vi "day2-1.vi"() -> ()   [LabVIEW 2021]
uses:
  <vilib>/Utility/file.llb/Read Delimited Spreadsheet (string).vi
panel:
  in  "Example":string="A Y\nB X\nC Z"
  in  "Example":bool
  out "Answer":i64=10624
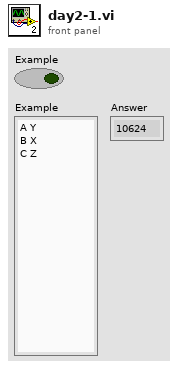
[diagram p1: front panel]
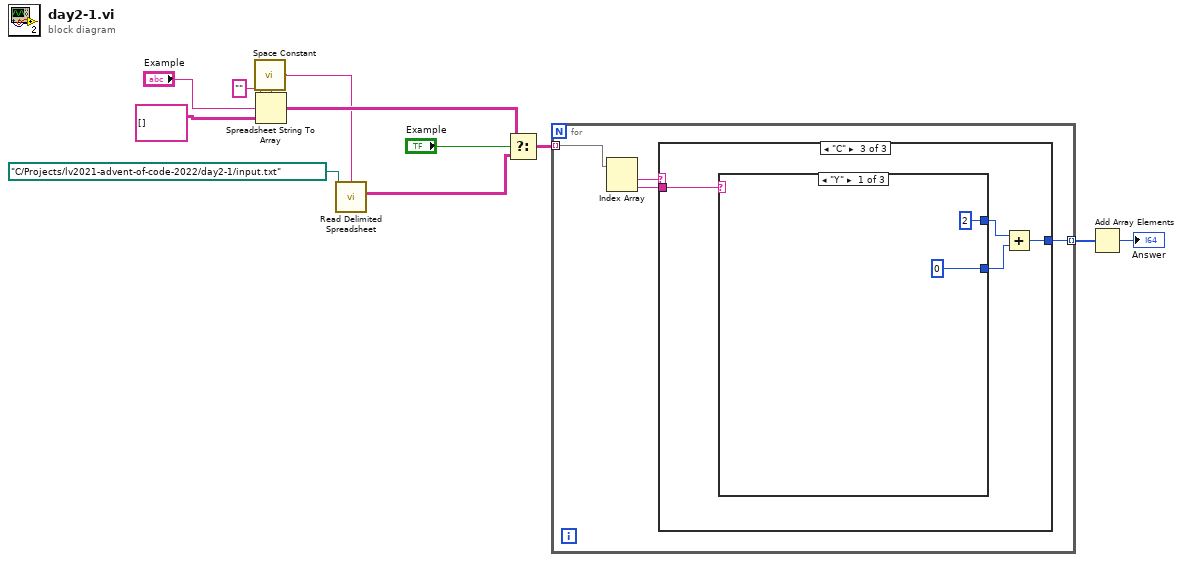
[diagram p0: block diagram]
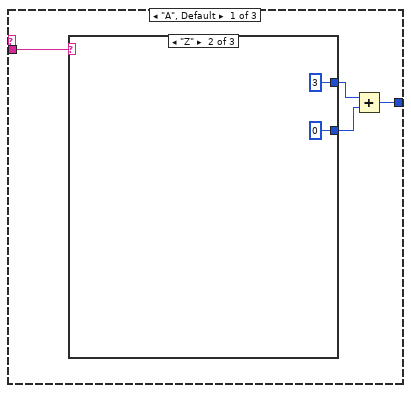
[diagram p2: hidden frame]
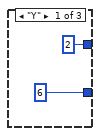
[diagram p3: hidden frame]
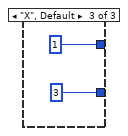
[diagram p4: hidden frame]
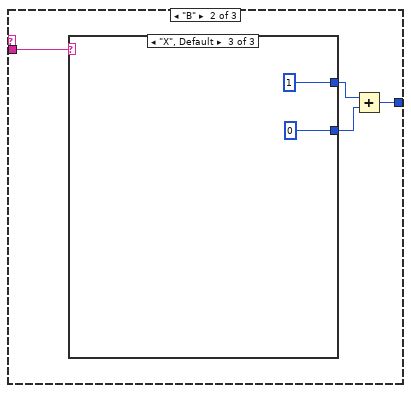
[diagram p5: hidden frame]
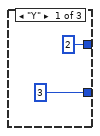
[diagram p6: hidden frame]
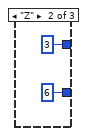
[diagram p7: hidden frame]
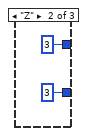
[diagram p8: hidden frame]
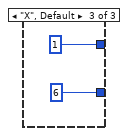
[diagram p9: hidden frame]
diagram:
  n1 = call <vilib>:"Space Constant.vi"() -> ("String"=w3:string)
  n2 = Spreadsheet String To Array(delimiter (Tab)=w3, format string="", spreadsheet string="Example", array type (2D Dbl)=string[][] [] ("t")) -> (array=w7:string[][])
  n3 = call-poly <vilib>:"Read Delimited Spreadsheet.vi"("file path (dialog if empty)"=path "C:/Projects/lv2021-advent-of-code-2022/day2-1/input.txt", "delimiter (\\t)"=w3) -> ("all rows"=w4:string[][])  [unwired: 8 in, 5 out]
  n4 = Select(t=w7, s="Example", f=w4) -> (s? t:f=w10:string[][])
  n5 = for {
    tunnel: w10 -> [w14] mode=indexing
    tunnel: [w12] -> w2 mode=indexing
    n6 = Index Array(array=w14) -> (element #1=w15:string, element #2=w13:string)  [unwired: 2 in]
    n7 = case shown="\"C\"" w15 {
      tunnel: w13 -> [w19 w29 w39]
      tunnel: [w16 w26 w36] -> w12
      frame "A", Default {
        n8 = case shown="\"Z\"" w19 {
          tunnel: [6 0 3] -> w17
          tunnel: [2 3 1] -> w18
          frame "Y" {
          }
          frame "Z" {
          }
          frame "X", Default {
          }
        }
        n9 = Add(x=w18, y=w17) -> (x+y=w16:i32)
      }
      frame "B" {
        n10 = case shown="\"X\", Default" w29 {
          tunnel: [3 6 0] -> w27
          tunnel: [2 3 1] -> w28
          frame "Y" {
          }
          frame "Z" {
          }
          frame "X", Default {
          }
        }
        n11 = Add(x=w28, y=w27) -> (x+y=w26:i32)
      }
      frame "C" {
        n12 = case shown="\"Y\"" w39 {
          tunnel: [0 3 6] -> w37
          tunnel: [2 3 1] -> w38
          frame "Y" {
          }
          frame "Z" {
          }
          frame "X", Default {
          }
        }
        n13 = Add(x=w38, y=w37) -> (x+y=w36:i32)
      }
    }
  }
  n14 = Add Array Elements(numeric array=w2) -> (sum=→"Answer":i32)
